vi "z bytes slice iterator next.vi"(8 "error in (no error)":errorcluster, 10 "slice":cluster{}, 11 "this_":cluster{}) -> (0 "error out":errorcluster, 1 "function return":bool, 2 "slice out":cluster{}, 3 "this_ out":cluster{})   [LabVIEW 2021, in "zenohc.lvlib"]
doc: "bool z_bytes_slice_iterator_next(struct z_bytes_slice_iterator_t *this_,\n struct z_view_slice_t *slice);"
uses:
  zenohc.lvlib
  zenohc.dll
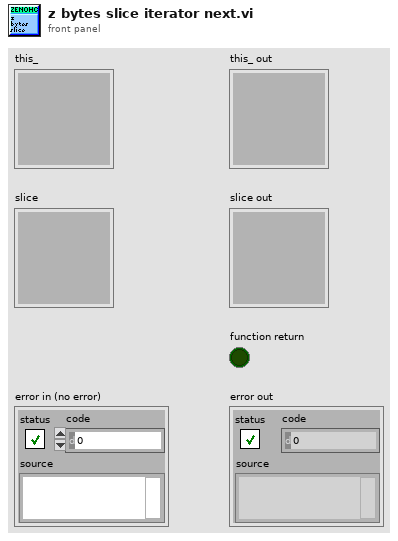
[diagram p1: front panel]
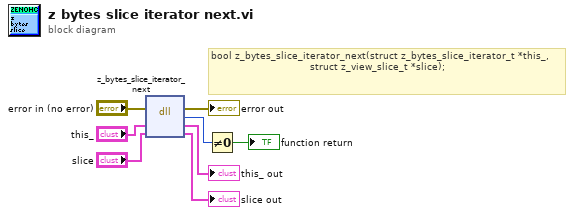
[diagram p0: block diagram]
diagram:
  # "bool z_bytes_slice_iterator_next(struct z_bytes_slice_iterator_t *this_,\n                                 struct z_view_slice_t *slice);"
  n1 = dll-call lib="D:/dev/zenoh_labview/zenohc/zenohc.*" fn="z_bytes_slice_iterator_next"(error in="error in (no error)", "this_"="this_", "slice"="slice") -> (error out=→"error out":errorcluster, w7:u8, "this_"=→"this_ out":cluster{}, "slice"=→"slice out":cluster{})  [unwired: 2 in, 1 out]
  n2 = Not Equal To 0?(x=w7) -> (x != 0?=→"function return":bool)
